vi "DRAMFIFO_Host.vi"() -> ()   [LabVIEW 2014]
uses:
  <vilib>/rvi/interface/nirviOpenFPGA/nirviOpenFPGA.xnode
  <vilib>/rvi/interface/nirviMethod/nirviMethod.xnode
  <vilib>/rvi/errors/niLvFpgaMergeErrorWithErrorCode.vi
  <vilib>/rvi/interface/nirviReadWriteControl/nirviReadWriteControl.xnode
  <instrlib>/_niInstr/Streaming/v1/Host/niInstr Streaming v1 Host.lvlib
  <instrlib>/_niInstr/Streaming/v1/Host/Public/Start Finite Stream.vi
  <vilib>/rvi/interface/nirviCloseFPGA/nirviCloseFPGA.xnode
  <instrlib>/_niInstr/Streaming/v1/Host/Public/Wait for Stream.vi
  <vilib>/FPGAPlugInAG/Dynamic/niLvFpga_ConfigureFifo_Dynamic.vi
  <vilib>/FPGAPlugInAG/Dynamic/niLvFpga_StartFifo_Dynamic.vi
  NiFpgaLv.dll
  <vilib>/Utility/error.llb/Error Cluster From Error Code.vi
  <vilib>/rvi/interface/Simulation/niFpgaSimulationCallBeginRW.vi
  <vilib>/rvi/errors/niLvFpgaAdjustHostInterfaceError.vi
  <vilib>/FPGAPlugInAG/Dynamic/niLvFpga_ReadFifo_Dynamic.vi
  <vilib>/FPGAPlugInAG/Dynamic/niLvFpga_Close_Dynamic.vi
  FPGA Bitfiles/DRAMFIFOTest_FPGATarget2_DRAMFPGA_xB81jlXoDQs.lvbitx
  DRAM FPGA.vi
  <vilib>/FPGAPlugInAG/PXIe-7975R/niLvFpga_Open_PXIe-7975R.vi
  <vilib>/rvi/interface/common/dynamic/niFpgaDynamicAddResources.vi
panel:
  in  "num samples":u64=1000
  in  "read grant time (clocks)":u16=100
  in  "write grant time (clocks)":u16=100
  out "error out":errorcluster
  in  "Stop Button":bool
  out "Waveform Graph":i16[](graph)
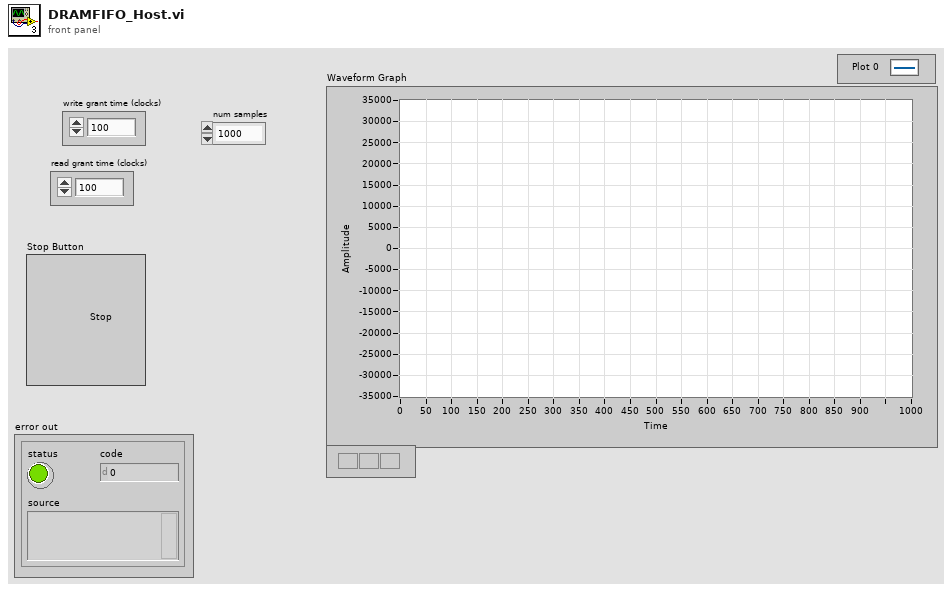
[diagram p1: front panel]
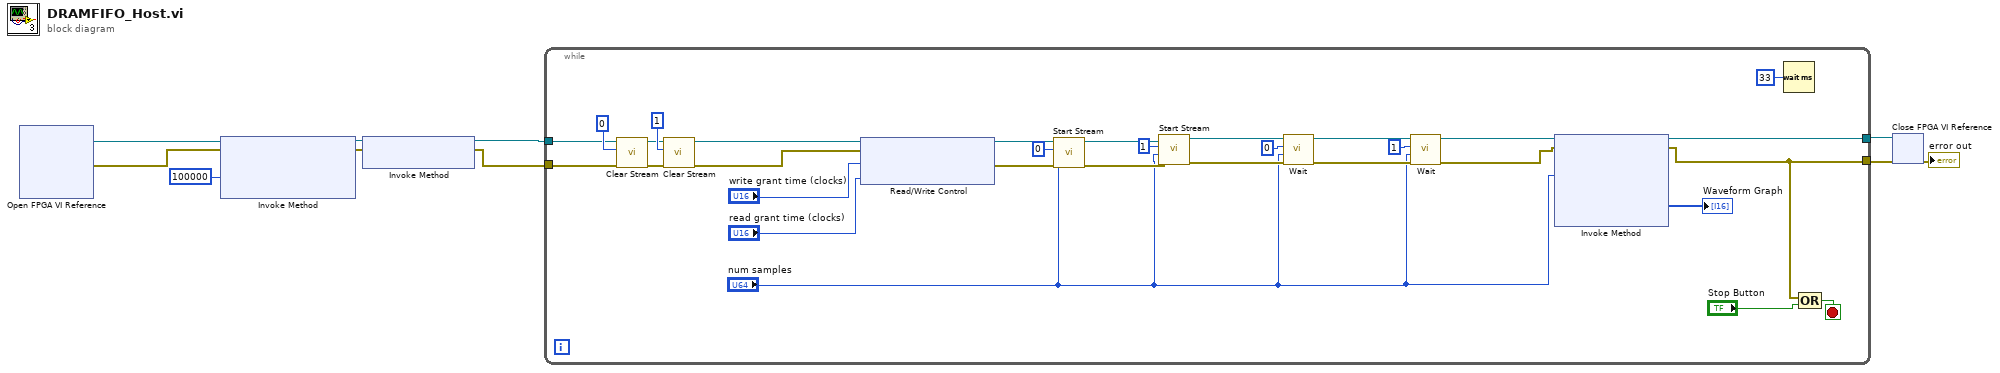
[diagram p0: block diagram]
diagram:
  n1 = xnode "Open FPGA VI Reference"() -> ("FPGA VI Reference Out"=w3:refnum<k20>, "error out"=w4:errorcluster)  [unwired: 2 in]
  n2 = xnode "Invoke Method"("FPGA VI Reference In"=w3, "error in"=w4, "Requested Depth"=u32 100000) -> ("FPGA VI Reference Out"=w10:refnum<k20>, "error out"=w9:errorcluster)  [unwired: 1 out]
  n3 = xnode "Invoke Method"("FPGA VI Reference In"=w10, "error in"=w9) -> ("FPGA VI Reference Out"=w2:refnum<k20>, "error out"=w1:errorcluster)
  n4 = while {
    tunnel: w2 -> [w16]
    tunnel: w1 -> [w15]
    tunnel: [w24] -> w7
    tunnel: [w23] -> w6
    stop <- w25 stop-if-true
    n5 = call <instrlib>:"Clear Stream.vi"("error in (no error)"=w15, "stream index"=0, "refnum in"=w16) -> ("error out"=w18:errorcluster, "refnum out"=w19:refnum<k20>)  [unwired: 7 in]
    n6 = call <instrlib>:"Clear Stream.vi"("error in (no error)"=w18, "stream index"=1, "refnum in"=w19) -> ("error out"=w13:errorcluster, "refnum out"=w14:refnum<k20>)  [unwired: 7 in]
    n7 = xnode "Read/Write Control"("FPGA VI Reference In"=w14, "error in"=w13, "write grant time (clocks)"="write grant time (clocks)", "read grant time (clocks)"="read grant time (clocks)") -> ("FPGA VI Reference Out"=w41:refnum<k20>, "error out"=w40:errorcluster)
    n8 = call-poly <instrlib>:"Start Stream.vi"("error in (no error)"=w40, "num samples"="num samples", "stream index"=0, "refnum in"=w41) -> ("error out"=w38:errorcluster, "refnum out"=w39:refnum<k20>)  [unwired: 6 in]
    n9 = call-poly <instrlib>:"Start Stream.vi"("error in (no error)"=w38, "num samples"="num samples", "stream index"=1, "refnum in"=w39) -> ("error out"=w21:errorcluster, "refnum out"=w22:refnum<k20>)  [unwired: 6 in]
    n10 = call-poly <instrlib>:"Wait.vi"("error in (no error)"=w21, "wait for samples transferred"="num samples", "stream index"=0, "refnum in"=w22) -> ("error out"=w33:errorcluster, "refnum out"=w34:refnum<k20>)  [unwired: 4 in, 2 out]
    n11 = call-poly <instrlib>:"Wait.vi"("error in (no error)"=w33, "wait for samples transferred"="num samples", "stream index"=1, "refnum in"=w34) -> ("error out"=w36:errorcluster, "refnum out"=w37:refnum<k20>)  [unwired: 4 in, 2 out]
    n12 = xnode "Invoke Method"("FPGA VI Reference In"=w37, "error in"=w36, "Number of Elements"="num samples") -> ("FPGA VI Reference Out"=w24:refnum<k20>, "error out"=w23:errorcluster, "Data"=→"Waveform Graph":i16[])  [unwired: 1 in, 1 out]
    n13 = Wait (ms)(milliseconds to wait=u32 33) -> ()  [unwired: 1 out]
    n14 = Compound Arithmetic op=OR(w23, "Stop Button") -> (w25:bool)
  }
  n15 = xnode "Close FPGA VI Reference"("FPGA VI Reference In"=w7, "error in"=w6) -> ("error out"=→"error out":errorcluster)
